vi "spring - find item.vi"(6 "indentation":i32=-1, 8 "error in (no error)":errorcluster, 9 "item index":i32=-1, 10 "primary itemstring to be found":string, 11 "tree data":T1[](array[typedef])) -> (0 "error out":errorcluster, 1 "son# (0=first)":i32=-1, 2 "parent tag":string, 3 "moved item's index":i32=-1)   [LabVIEW 2014]
uses:
  spring - node data.ctl
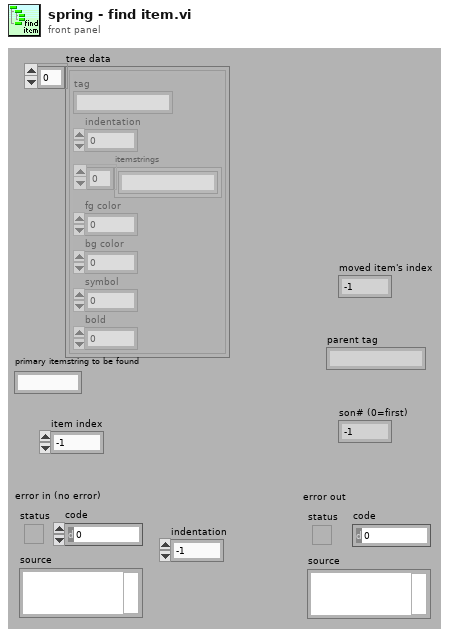
[diagram p1: front panel]
types:
  T1 = typedef "spring - node data.ctl" = cluster{"tag":string, "indentation":i32, "itemstrings":string[], "fg color":u32, "bg color":u32, "symbol":u32, "bold":u32}
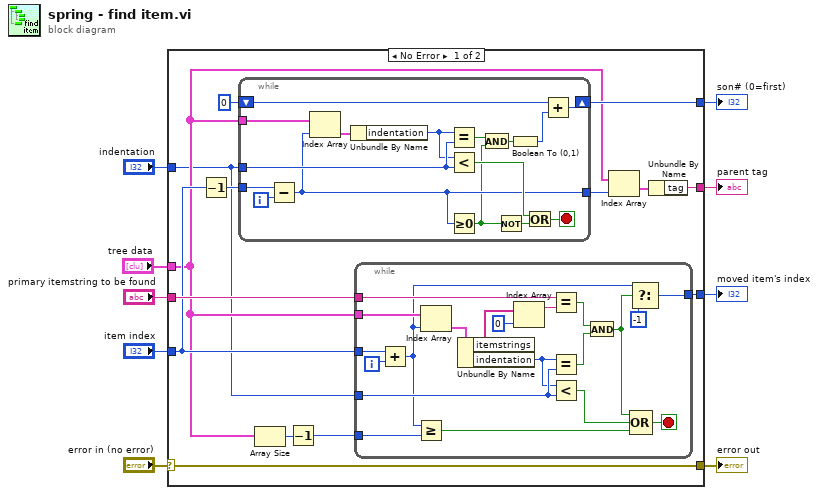
[diagram p0: block diagram]
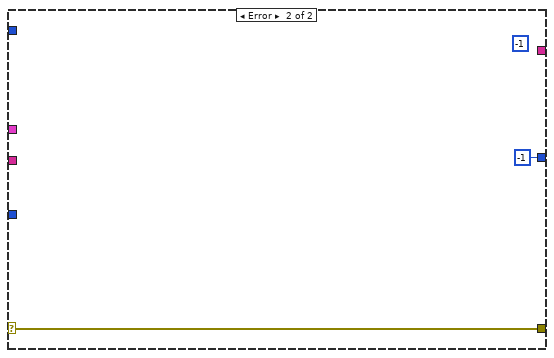
[diagram p2: hidden frame]
diagram:
  n1 = case shown="No Error" "error in (no error)" {
    selector: "error in (no error)" -> [w20 w61]
    tunnel: [w20 w61] -> w9
    tunnel: "tree data" -> [w15 _]
    tunnel: "item index" -> [w17 _]
    tunnel: "primary itemstring to be found" -> [w22 _]
    tunnel: [w21 -1 ("f")] -> w5
    tunnel: "indentation" -> [w10 _]
    tunnel: [w16 _] -> w2
    tunnel: [w13 _] -> w1
    frame No Error {
      n2 = Decrement(x=w17) -> (x-1=w18:i32)
      n3 = while {
        tunnel: w15 -> [w36]
        tunnel: w10 -> [w39]
        tunnel: w18 -> [w37]
        shift-right: [w35] -> w16
        shift-left: 0 -> [w31]
        tunnel: [w28] -> w11
        i -> [w38]
        stop <- w34 stop-if-true
        n4 = Subtract(x=w37, y=w38) -> (x-y=w28:i32)
        n5 = Index Array(array=w36, index=w28) -> (element=w25:T1)
        n6 = Unbundle By Name(w25) -> ("indentation"=w24:i32)
        n7 = Equal?(x=w24, y=w39) -> (x = y?=w30:bool)
        n8 = Less?(x=w24, y=w39) -> (x < y?=w33:bool)
        n9 = Greater Or Equal To 0?(x=w28) -> (x >= 0?=w27:bool)
        n10 = And(x=w30, y=w27) -> (x .and. y?=w29:bool)
        n11 = Not(x=w27) -> (.not. x?=w26:bool)
        n12 = Boolean To (0,1)(Boolean=w29) -> (0, 1=w32:i16)
        n13 = Or(x=w33, y=w26) -> (x .or. y?=w34:bool)
        n14 = Add(x=w31, y=w32) -> (x+y=w35:i32)
      }
      n15 = Array Size(array=w15) -> (size(s)=w19:i32)
      n16 = Decrement(x=w19) -> (x-1=w23:i32)
      n17 = while {
        tunnel: w15 -> [w56]
        tunnel: w10 -> [w59]
        tunnel: w17 -> [w57]
        tunnel: w23 -> [w53]
        tunnel: w22 -> [w51]
        tunnel: [w45] -> w21
        i -> [w58]
        stop <- w54 stop-if-true
        n18 = Add(x=w57, y=w58) -> (x+y=w47:i32)
        n19 = Greater Or Equal?(x=w47, y=w53) -> (x >= y?=w52:bool)
        n20 = Index Array(array=w56, index=w47) -> (element=w44:T1)
        n21 = Unbundle By Name(w44) -> ("itemstrings"=w42:string[], "indentation"=w43:i32)
        n22 = Index Array(array=w42, index=0) -> (element=w40:string)
        n23 = Equal?(x=w51, y=w40) -> (x = y?=w49:bool)
        n24 = Equal?(x=w43, y=w59) -> (x = y?=w50:bool)
        n25 = Less?(x=w43, y=w59) -> (x < y?=w55:bool)
        n26 = And(x=w49, y=w50) -> (x .and. y?=w48:bool)
        n27 = Select(t=w47, s=w48, f=-1) -> (s? t:f=w45:i32)
        n28 = Compound Arithmetic op=OR(w48, w55, w52) -> (w54:bool)
      }
      n29 = Index Array(array=w15, index=w11) -> (element=w14:T1)
      n30 = Unbundle By Name(w14) -> ("tag"=w13:string)
    }
    frame Error {
      (unwired) -1
    }
  }
  "error out" <- w9
  "moved item's index" <- w5
  "son# (0=first)" <- w2
  "parent tag" <- w1
